vi "Beampointing get motor position tcp.vi"(7 "Active CCD":i32, 8 "error in (no error)":errorcluster, 11 "dev variable alias Motors X":string[][](array[string])) -> (0 "error out":errorcluster, 3 "value":dbl)   [LabVIEW 2020]
panel:
  out "variable value":string
  out "timed out":bool
  out "Variable name":string
  out "Device name":string
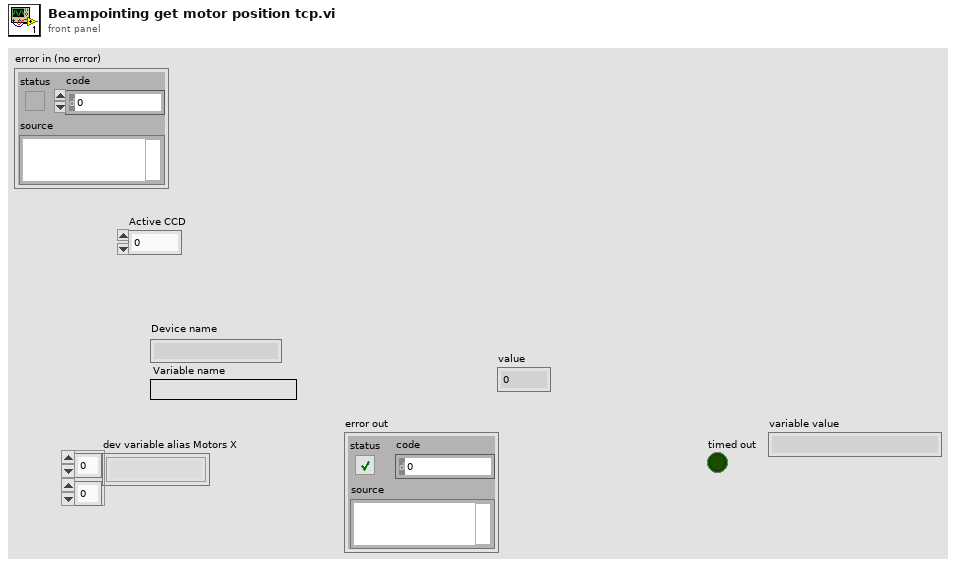
[diagram p1: front panel]
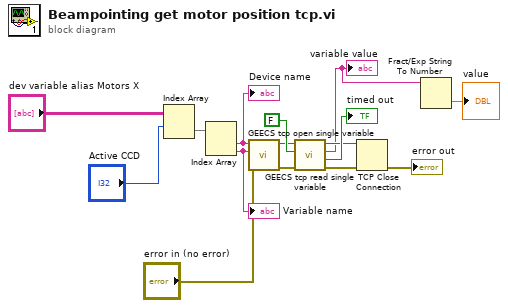
[diagram p0: block diagram]
diagram:
  n1 = Index Array(array="dev variable alias Motors X", index (row)="Active CCD") -> (element=w6:string[])  [unwired: 1 in]
  n2 = Index Array(array=w6) -> (element #1=w5:string, element #2=w4:string)  [unwired: 2 in]
  "Device name" <- w5
  "Variable name" <- w4
  n3 = call "GEECS tcp open single variable.vi"("error in (no error)"="error in (no error)", "Variable name"=w4, "Device name"=w5) -> ("error out"=w11:errorcluster, "TCP Network Connection out"=w12:refnum<k5>)  [unwired: 6 in, 1 out]
  n4 = call "GEECS tcp read single variable.vi"("error in (no error)"=w11, "clear buffer after read"=FALSE, "TCP Network Connection in"=w12) -> ("error out"=w10:errorcluster, "timed out"=→"timed out":bool, "variable value"=w2:string, "TCP Network Connection out"=w9:refnum<k5>)  [unwired: 5 in]
  "variable value" <- w2
  n5 = TCP Close Connection(connection ID=w9, error in (no error)=w10) -> (error out=→"error out":errorcluster)  [unwired: 1 in, 1 out]
  n6 = Fract/Exp String To Number(string=w2) -> (number=→"value":dbl)  [unwired: 3 in, 1 out]
